vi "gen_stepfunc.vi"(8 "error in (no error)":errorcluster, 11 "TrajectoryAK101022Resonance in":refnum<class "TrajectoryAK101022Resonance.lvclass">) -> (0 "error out":errorcluster, 2 "z-Points Array":dbl[](array[numeric]), 3 "TrajectoryAK101022Resonance out":refnum<class "TrajectoryAK101022Resonance.lvclass">)   [LabVIEW 2010, in "TrajectoryAK101022Resonance.lvclass"]
uses:
  TrajectoryAK101022Resonance.lvclass
  TrajectoryAK101022Resonance.lvclass/TrajectoryAK101022Resonance.ctl
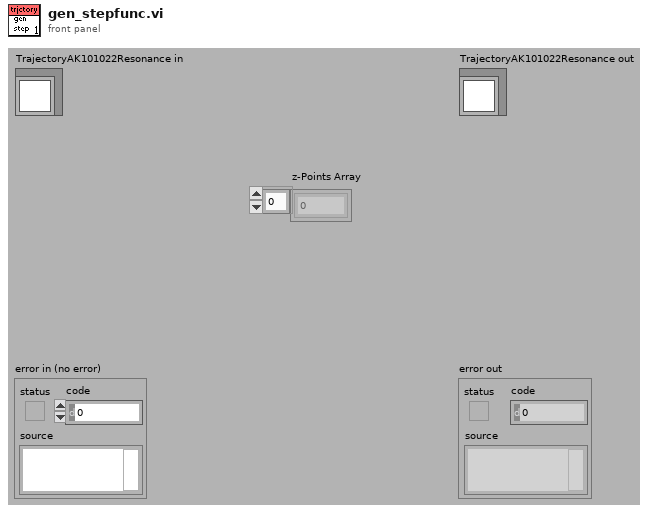
[diagram p1: front panel]
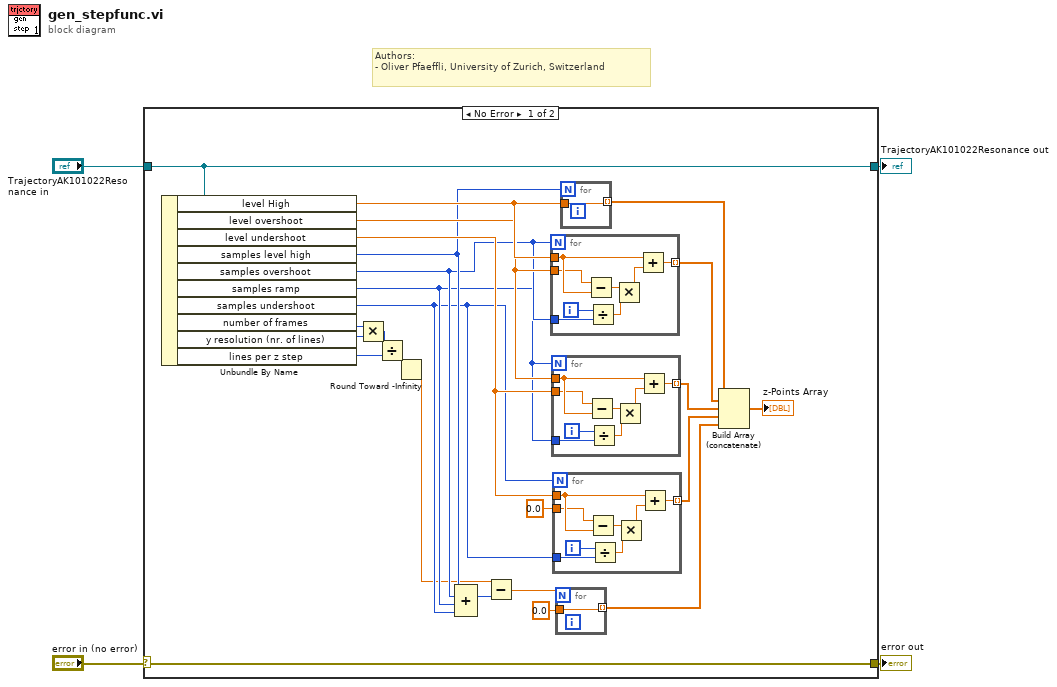
[diagram p0: block diagram]
diagram:
  # "Authors: \n- Oliver Pfaeffli, University of Zurich, Switzerland"
  n1 = case shown="No Error" "error in (no error)" {
    selector: "error in (no error)" -> [w29 w57]
    tunnel: [w29 w57] -> w3
    tunnel: [w28 w56] -> w1
    tunnel: "TrajectoryAK101022Resonance in" -> [w28 w56]
    frame No Error {
      n2 = Unbundle By Name(w28) -> ("level High"=w27:dbl, "level overshoot"=w26:dbl, "level undershoot"=w25:dbl, "samples level high"=w23:u16, "samples overshoot"=w22:u16, "samples ramp"=w21:u16, "samples undershoot"=w11:u16, "number of frames"=w10:i32, "y resolution (nr. of lines)"=w9:i32, "lines per z step"=w7:i32)
      n3 = Multiply(x=w10, y=w9) -> (x*y=w8:i32)
      n4 = Divide(x=w8, y=w7) -> (x/y=w6:dbl)
      n5 = Round Toward -Infinity(1:w6) -> (0:w5:dbl)
      n6 = Compound Arithmetic op=ADD(w23, w22, w21, w11) -> (w20:u16)
      n7 = Subtract(x=w5, y=w20) -> (x-y=w19:dbl)
      n8 = for {
        N: w22 -> [_]
        tunnel: w27 -> [w54]
        tunnel: w26 -> [w53]
        tunnel: w22 -> [w51]
        tunnel: [w47] -> w16 mode=indexing
        i -> [w52]
        n9 = Subtract(x=w53, y=w54) -> (x-y=w50:dbl)
        n10 = Divide(x=w52, y=w51) -> (x/y=w49:dbl)
        n11 = Multiply(x=w50, y=w49) -> (x*y=w48:dbl)
        n12 = Add(x=w54, y=w48) -> (x+y=w47:dbl)
      }
      n13 = for {
        N: w21 -> [_]
        tunnel: w26 -> [w46]
        tunnel: w25 -> [w45]
        tunnel: w21 -> [w43]
        tunnel: [w39] -> w15 mode=indexing
        i -> [w44]
        n14 = Subtract(x=w45, y=w46) -> (x-y=w42:dbl)
        n15 = Divide(x=w44, y=w43) -> (x/y=w41:dbl)
        n16 = Multiply(x=w42, y=w41) -> (x*y=w40:dbl)
        n17 = Add(x=w46, y=w40) -> (x+y=w39:dbl)
      }
      n18 = for {
        N: w11 -> [_]
        tunnel: w25 -> [w38]
        tunnel: 0.0 ("LinesLevel undershoot") -> [w37]
        tunnel: w11 -> [w35]
        tunnel: [w31] -> w14 mode=indexing
        i -> [w36]
        n19 = Subtract(x=w37, y=w38) -> (x-y=w34:dbl)
        n20 = Divide(x=w36, y=w35) -> (x/y=w33:dbl)
        n21 = Multiply(x=w34, y=w33) -> (x*y=w32:dbl)
        n22 = Add(x=w38, y=w32) -> (x+y=w31:dbl)
      }
      n23 = for {
        N: w19 -> [_]
        tunnel: [w30] -> w13 mode=indexing
        tunnel: 0.0 ("LinesLevel undershoot") -> [w30]
      }
      n24 = for {
        N: w23 -> [_]
        tunnel: [w55] -> w17 mode=indexing
        tunnel: w27 -> [w55]
      }
      n25 = Build Array (concatenate)(w17, w16, w15, w14, w13) -> (→"z-Points Array":dbl[])
    }
    frame Error {
    }
  }
  "error out" <- w3
  "TrajectoryAK101022Resonance out" <- w1
